vi "Paint Largest Bounding Box.vi"(10 "Border Width":dbl=2.0 format="%#_13g", 11 "Particle Reports (Pixels)":T1(array[cluster]) {"Orientation" format="%.2f"; "Dimensions"."Height" format="%.2f"; "Dimensions"."Width" format="%.2f"; "Center of Mass"."Y" format="%.2f"; "Center of Mass"."X" format="%.2f"; "Bounding Rect"."Bottom" format="%.2f"; "Bounding Rect"."Right" format="%.2f"; "Bounding Rect"."Top" format="%.2f"; "Bounding Rect"."Left" format="%.2f"; "Number of Holes" format="%.2f"; "Area" format="%.2f"}) -> (2 "Bounding Box":cluster{dbl, dbl, dbl, dbl, dbl}, 3 "Dimensions":cluster{dbl, dbl})   [LabVIEW 2018]
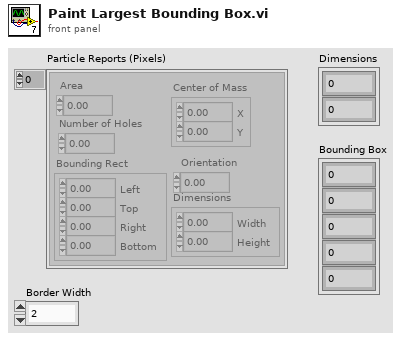
[diagram p1: front panel]
types:
  T1 = cluster{"Area":dbl, "Number of Holes":dbl, "Bounding Rect":cluster{"Left":dbl, "Top":dbl, "Right":dbl, "Bottom":dbl}, "Center of Mass":cluster{"X":dbl, "Y":dbl}, "Orientation":dbl, "Dimensions":cluster{"Width":dbl, "Height":dbl}}[]
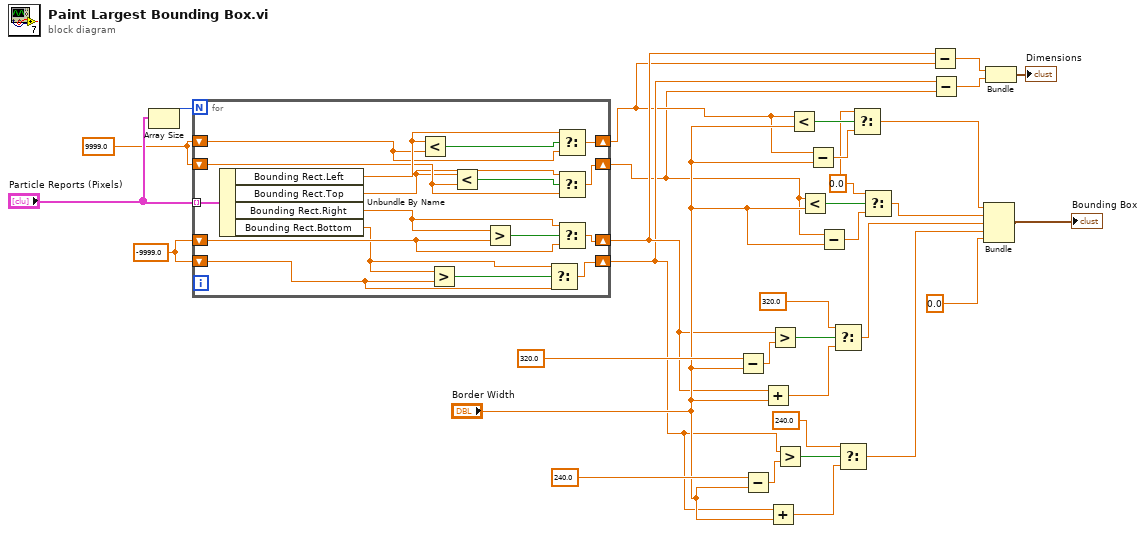
[diagram p0: block diagram]
diagram:
  w1 = 0.0
  w26 = -9999.0
  w27 = 9999.0
  n1 = Array Size(array="Particle Reports (Pixels)") -> (size(s)=w28:i32)
  n2 = for {
    N: w28 -> [_]
    tunnel: "Particle Reports (Pixels)" -> [w50] mode=indexing
    shift-right: [w46] -> w5
    shift-left: w27 -> [w47]
    shift-right: [w43] -> w4
    shift-left: w27 -> [w44]
    shift-right: [w38] -> w7
    shift-left: w26 -> [w39]
    shift-right: [w34] -> w6
    shift-left: w26 -> [w36]
    n3 = Unbundle By Name(w50) -> ("Bounding Rect.Left"=w48:dbl, "Bounding Rect.Top"=w42:dbl, "Bounding Rect.Right"=w40:dbl, "Bounding Rect.Bottom"=w35:dbl)
    n4 = Less?(x=w48, y=w47) -> (x < y?=w49:bool)
    n5 = Greater?(x=w35, y=w36) -> (0:w37:bool)
    n6 = Less?(x=w42, y=w44) -> (x < y?=w45:bool)
    n7 = Greater?(x=w40, y=w39) -> (0:w41:bool)
    n8 = Select(t=w35, s=w37, f=w36) -> (s? t:f=w34:dbl)
    n9 = Select(t=w48, s=w49, f=w47) -> (s? t:f=w46:dbl)
    n10 = Select(t=w42, s=w45, f=w44) -> (s? t:f=w43:dbl)
    n11 = Select(t=w40, s=w41, f=w39) -> (s? t:f=w38:dbl)
  }
  n12 = Subtract(x=320.0, y="Border Width") -> (x-y=w16:dbl)
  n13 = Subtract(x=240.0, y="Border Width") -> (x-y=w14:dbl)
  n14 = Add(x=w7, y="Border Width") -> (x+y=w20:dbl)
  n15 = Add(x=w6, y="Border Width") -> (x+y=w13:dbl)
  n16 = Greater?(x=w7, y=w16) -> (0:w21:bool)
  n17 = Greater?(x=w6, y=w14) -> (0:w12:bool)
  n18 = Less?(x=w5, y="Border Width") -> (x < y?=w25:bool)
  n19 = Less?(x=w4, y="Border Width") -> (x < y?=w22:bool)
  n20 = Subtract(x=w5, y="Border Width") -> (x-y=w24:dbl)
  n21 = Subtract(x=w4, y="Border Width") -> (x-y=w23:dbl)
  n22 = Select(t=320.0 ("x"), s=w21, f=w20) -> (s? t:f=w15:dbl)
  n23 = Select(t=240.0 ("x"), s=w12, f=w13) -> (s? t:f=w11:dbl)
  n24 = Select(t=w1, s=w25, f=w24) -> (s? t:f=w18:dbl)
  n25 = Select(t=w1, s=w22, f=w23) -> (s? t:f=w19:dbl)
  n26 = Subtract(x=w7, y=w5) -> (x-y=w29:dbl)
  n27 = Subtract(x=w6, y=w4) -> (x-y=w30:dbl)
  n28 = Bundle(w18, w19, "x"=w15, "x"=w11, 0.0) -> (→"Bounding Box":cluster{dbl, dbl, "x":dbl, "x":dbl, dbl})  [unwired: 1 in]
  n29 = Bundle(w29, w30) -> (→"Dimensions":cluster{dbl, dbl})  [unwired: 1 in]
